vi "Strip apostrophe.vi"   [LabVIEW 2019]
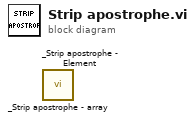
[diagram p0: block diagram]
diagram:
  n1 = call "_Strip apostrophe - array.vi"() -> ()  [unwired: 11 in, 1 out]
  n2 = call "_Strip apostrophe - Element.vi"() -> ()  [unwired: 11 in, 1 out]
